vi "Cycle Duration Post Sub Steps types.vi"(10 "Cycle Duration Data in":T1, 11 "Sequence Context In":refnum<k7>) -> (0 "error out":errorcluster, 2 "Cycle Duration Data out":T1, 3 "Report Text":string)   [LabVIEW 2023, in "LTT_TeststandSteptypes.lvlib"]
uses:
  LTT_TeststandSteptypes.lvlib
  Control/Cycle Duration Data.ctl
  Control/Cycle Duration Selection.ctl
  HardwareAbstractionLayer_LVOOP/Report/Report_class/Control/Action FGV.ctl
  HardwareAbstractionLayer_LVOOP/Report/Report_class/Control/All Log Details.ctl
  HardwareAbstractionLayer_LVOOP/Report/Report_class/Control/UUT Test Info.ctl
  HardwareAbstractionLayer_LVOOP/Report/Report_class/Control/FE FRAME LOG.ctl
  HardwareAbstractionLayer_LVOOP/Report/Report_class/Control/FF FRAME LOG.ctl
  HardwareAbstractionLayer_LVOOP/Report/Report_class/Control/LIMIT TABLE.ctl
  HardwareAbstractionLayer_LVOOP/Report/Report_class/Control/ERROR LOG APPEND.ctl
  HardwareAbstractionLayer_LVOOP/Report/Report_class/Control/ERROR LOG.ctl
  HardwareAbstractionLayer_LVOOP/Report/Report_class/Control/FA FRAME LOG.ctl
  HardwareAbstractionLayer_LVOOP/Report/Report_class/Control/TEST RESULT LOG APPEND.ctl
  HardwareAbstractionLayer_LVOOP/Report/Report_class/Control/TEST RESULT LOG.ctl
  HardwareAbstractionLayer_LVOOP/Report/Report_class/Control/SYSTEM LOG.ctl
  HardwareAbstractionLayer_LVOOP/Report/Report_class/Control/Temperature LOG.ctl
  HardwareAbstractionLayer_LVOOP/Report/Report_class/Control/POWER STATUS.ctl
  HardwareAbstractionLayer_LVOOP/Report/Report_class/Control/CYCLE_DURATION_LOG.ctl
  HardwareAbstractionLayer_LVOOP/Database/SQL Public VI/Control/DB Options.ctl
  HardwareAbstractionLayer_LVOOP/Database/Database.lvclass
  HardwareAbstractionLayer_LVOOP/Report/Report_class/Report.lvclass
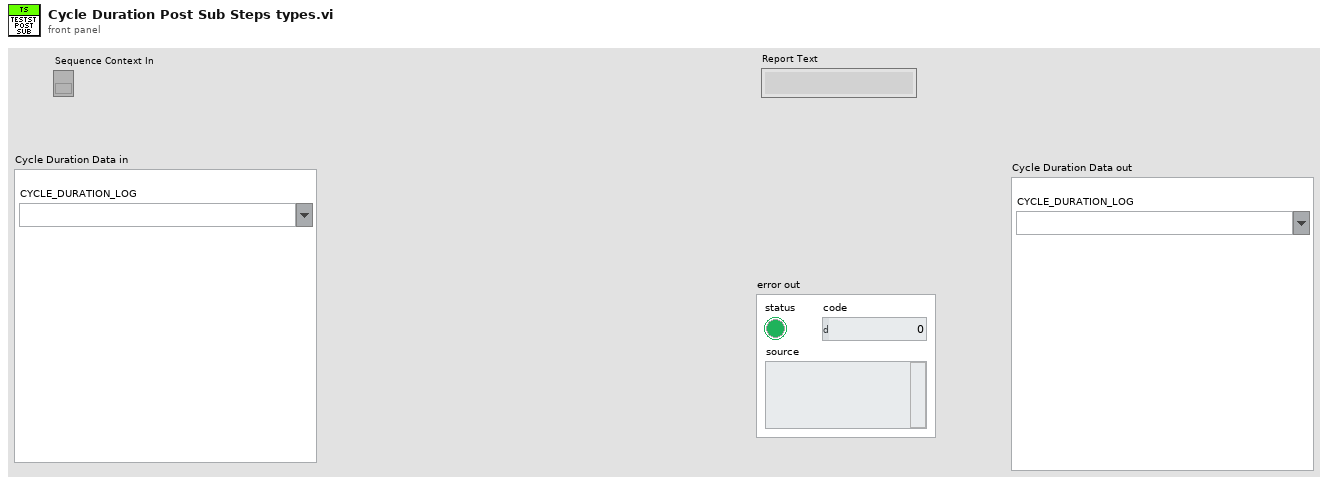
[diagram p1: front panel]
types:
  T1 = typedef "LTT_TeststandSteptypes.lvlib/Cycle Duration Data.ctl" = cluster{"CYCLE_DURATION_LOG":T2}
  T2 = typedef "LTT_TeststandSteptypes.lvlib/Cycle Duration Selection.ctl" = string
  T3 = typedef "HardwareAbstractionLayer_LVOOP.lvlib/Report.lvclass/Action FGV.ctl" = enum16{"Init", "Set Project Name", "Set Product Name", "Set Product Varient", "Set Test Name", "Set Test Phase", "Set Test Description", "Set Temp Chamber Name", "Set Cycle Duration", "Set Current Cycle Number", "Set Schema", "Set Total No Of Cycle", "Set Current Test Mode", "Set All Data", "Get All Data"}
  T4 = typedef "HardwareAbstractionLayer_LVOOP.lvlib/Report.lvclass/Result FGV Data.ctl" = cluster{"Project Name":string, "Product Name":string, "Product Varient":string, "Test Name":string, "Test Phase":string, "Test Description":string, "Temp Chamber Name":string, "Schema":string, "Total No of Cycles":u32, "Current Cycle Number":u32, "Cycle Duration":u32, "Current Test Mode":string}
  T5 = typedef "HardwareAbstractionLayer_LVOOP.lvlib/Report.lvclass/All Log Details.ctl" = cluster{"UUT_TEST_INFO":T6, "FE_FRAME_LOG":T7, "FF_FRAME_LOG":T8, "LIMIT_TABLE":T9, "ERROR LOG Append":T10, "FA_FRAME_LOG":T12, "Socket No":u16, "TEST RESULT LOG Append":T13, "SYSTEM_LOG":T15, "Temperature log":T16, "POWER_STATUS":T17, "CYCLE_DURATION_LOG":T18}
  T6 = typedef "HardwareAbstractionLayer_LVOOP.lvlib/Report.lvclass/UUT Test Info.ctl" = cluster{"ID":string, "STATION_ID":string, "TEST_SOCKET_INDEX":string, "UUT_SERIAL_NUMBER":string, "TSW_VER":string, "VAL_SW_VER":string, "PROJECT_NAME":string, "PRODUCT_NAME":string, "PRODUCT_VARIANT":string, "TEST_NAME":string, "TEST_PHASE":string, "TEST_DESCRIPTION":string, "TEMP_CHAMBER_NAME":string, "START_DATE_TIME":string, "STOP_DATE_TIME ":string, "START_CYCLE_COUNT":string, "STOP_CYCLE_COUNT":string, "EXECUTION_TIME":string, "UUT_STATUS":string, "UUT_ERROR_CODE":string, "UUT_ERROR_MESSAGE":string, "TEST_SEQUENCE":string}
  T7 = typedef "HardwareAbstractionLayer_LVOOP.lvlib/Report.lvclass/FE FRAME LOG.ctl" = cluster{"ID":string, "UUT_TEST_INFO":string, "DATE_TIME":string, "CYCLE_NUMBER":string, "TEST_MODE":string, "CHAMBER_TEMP":string, "CAN_FRAME_RX":string, "Test Mode":u32, "LV_PPS_VOLTAGE":string, "LV_PPS_CURRENT":string, "HV_PPS_VOLTAGE":string, "HV_PPS_CURRENT":string, "SOCKET_NUMBER":string, "CAN_FRAME_RX_NO_OFF_BYTE":string}
  T8 = typedef "HardwareAbstractionLayer_LVOOP.lvlib/Report.lvclass/FF FRAME LOG.ctl" = cluster{"ID":string, "UUT_TEST_INFO":string, "DATE_TIME":string, "CYCLE_NUMBER":string, "TEST_MODE":string, "CAN_FRAME_RX":string, "CHAMBER_TEMP":string, "TestMode":u32, "SOCKET_NUMBER":string, "CAN_FRAME_RX_NO_OFF_BYTE":string}
  T9 = typedef "HardwareAbstractionLayer_LVOOP.lvlib/Report.lvclass/LIMIT TABLE.ctl" = cluster{"ID":string, "PRODUCT_NAME":string, "PRODUCT_VARIANT":string, "TEST_MODE":string, "PARAMETER_NAME":string, "COMPARISON_TYPE":string, "LOW_LIMIT":string, "HIGH_LIMIT":string, "UNIT":string, "ERROR_MESSSAGE":string, "SEVERITY":string}
  T10 = typedef "HardwareAbstractionLayer_LVOOP.lvlib/Report.lvclass/ERROR LOG APPEND.ctl" = T11[]
  T11 = typedef "HardwareAbstractionLayer_LVOOP.lvlib/Report.lvclass/ERROR LOG.ctl" = cluster{"ID":string, "UUT_TEST_INFO":string, "DATE_TIME":string, "CYCLE_NUMBER":string, "TEST_MODE":string, "SIGNAL_NAME":string, "SIGNAL_VALUE":string, "UNIT":string, "COMPARISON_VALUE":string, "ERROR_MESSAGE":string, "FRAME_TYPE":string, "LIMITID":string, "SOCKET_NUMBER":string}
  T12 = typedef "HardwareAbstractionLayer_LVOOP.lvlib/Report.lvclass/FA FRAME LOG.ctl" = cluster{"UUT_TEST_INFO":string, "CAN_FRAME_RX":string, "CAN_FRAME_RX_NO_OFF_BYTE":string}
  T13 = typedef "HardwareAbstractionLayer_LVOOP.lvlib/Report.lvclass/TEST RESULT LOG APPEND.ctl" = T14[]
  T14 = typedef "HardwareAbstractionLayer_LVOOP.lvlib/Report.lvclass/TEST RESULT LOG.ctl" = cluster{"ID":string, "UUT_TEST_INFO":string, "DATE_TIME":string, "CYCLE_NUMBER":string, "TEST_MODE":string, "SIGNAL_NAME":string, "SIGNAL_VALUE":string, "COMPARISON_VALUE":string, "ERROR_MESSAGE":string, "FRAME_TYPE":string, "LIMITID":string, "TEST_RESULT":string, "SOCKET_NUMBER":string}
  T15 = typedef "HardwareAbstractionLayer_LVOOP.lvlib/Report.lvclass/SYSTEM LOG.ctl" = cluster{"ID ":string, "DATE_TIME":string, "CYCLE_NUMBER":string, "TEST_MODE":string, "ERROR_MESSAGE":string}
  T16 = typedef "HardwareAbstractionLayer_LVOOP.lvlib/Report.lvclass/Temperature LOG.ctl" = cluster{"TEST_MODE":string, "CYCLE_NUMBER":string, "TEMPERATURE":cluster{"LV_PPS_TEMPERATURE":dbl, "HV_PPS1_TEMPERATURE":dbl, "HV_PPS2_TEMPERATURE":dbl, "HV_PPS3_TEMPERATURE":dbl, "HV_PPS4_TEMPERATURE":dbl, "HV_PPS5_TEMPERATURE":dbl, "HV_PPS6_TEMPERATURE":dbl, "CHAMBER_TEMPERATURE":dbl, "LOAD_U1_TEMPERATURE":dbl, "LOAD_V1_TEMPERATURE":dbl, "LOAD_W1_TEMPERATURE":dbl, "LOAD_U2_TEMPERATURE":dbl, "LOAD_V2_TEMPERATURE":dbl, "LOAD_W2_TEMPERATURE":dbl, "LOAD_U3_TEMPERATURE":dbl, "LOAD_V3_TEMPERATURE":dbl, "LOAD_W3_TEMPERATURE":dbl}, "Temperature Inrange":cluster{"LVPPS_Trip?":bool, "HVPPS1_Trip?":bool, "HVPPS2_Trip?":bool, "HVPPS3_Trip?":bool, "HVPPS4_Trip?":bool, "HVPPS5_Trip?":bool, "HVPPS6_Trip?":bool, "Chamber_Trip?":bool}}
  T17 = typedef "HardwareAbstractionLayer_LVOOP.lvlib/Report.lvclass/POWER STATUS.ctl" = cluster{"TEST_MODE":string, "CYCLE_NUMBER":string, "TYPE_POWER":string, "STATE":string}
  T18 = typedef "HardwareAbstractionLayer_LVOOP.lvlib/Report.lvclass/CYCLE_DURATION_LOG.ctl" = cluster{"CYCLE_NUMBER":string}
  T19 = typedef "HardwareAbstractionLayer_LVOOP.lvlib/Database.lvclass/DB Options.ctl" = enum16{"Init", "Select Data", "Insert Data", "Update Data", "Delete Data", "Execute Query", "Create Schema", "Create Table", "List Tables", "List Columns", "Close"}
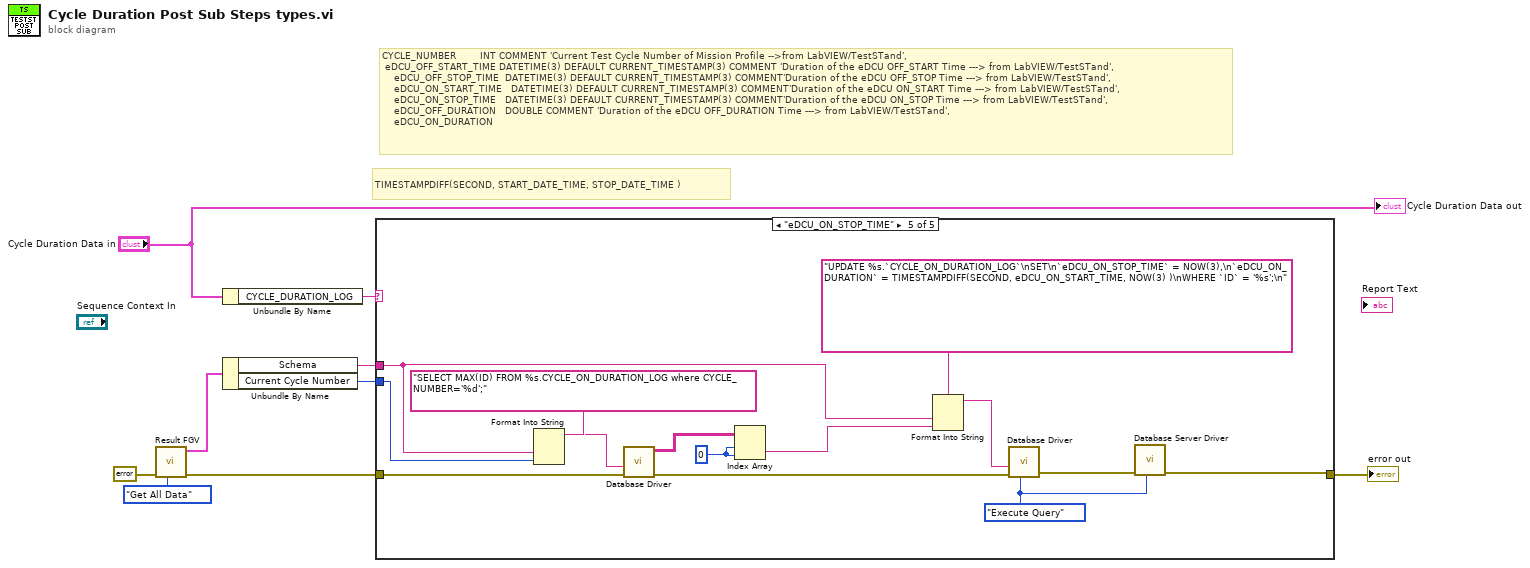
[diagram p0: block diagram]
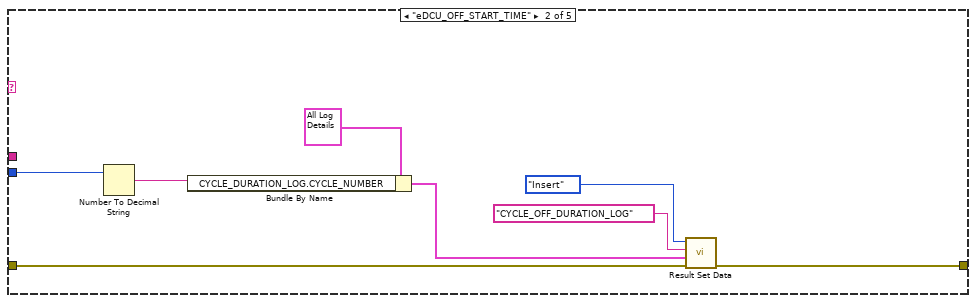
[diagram p3: hidden frame]
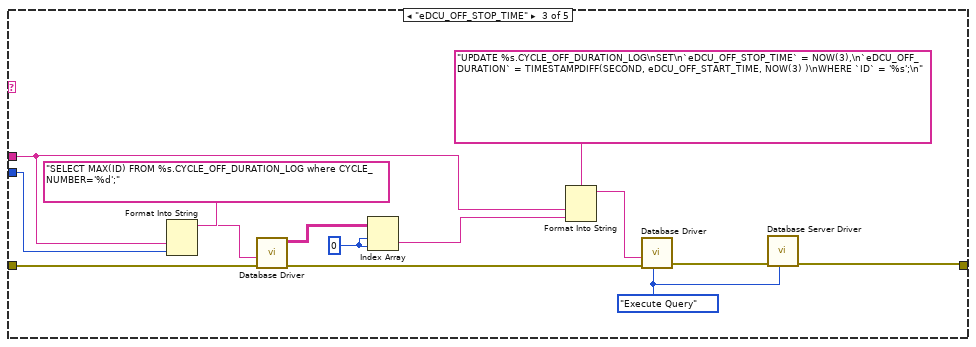
[diagram p4: hidden frame]
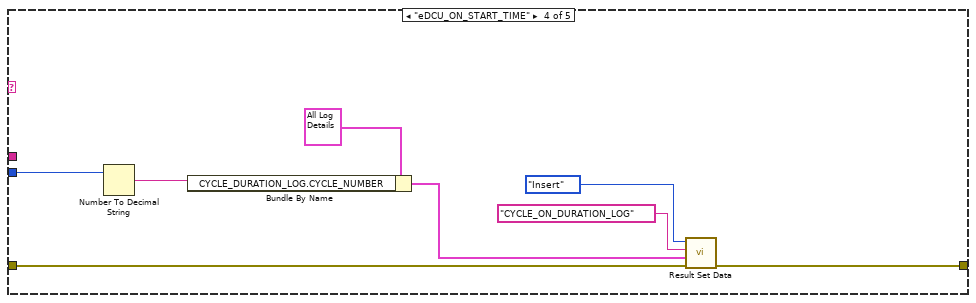
[diagram p5: hidden frame]
diagram:
  # "CYCLE_NUMBER        INT COMMENT 'Current Test Cycle Number of Mission Profile -->from LabVIEW/TestSTand',\n\teDCU_OFF_START_TIME DATETIME(3) DEFAULT CURRENT_TIMESTAMP(3) COMMENT 'Duration of the eDCU OFF_START Time ---> from LabVIEW/TestSTand',\n    eDCU_OFF_STOP_TIME  DATETIME(3) DEFAULT CURRENT_TIMESTAMP(3) COMMENT'Duration of the eDCU OFF_STOP Time ---> from LabVIEW/TestSTand',\n    eDCU_ON_START_TIME   DATETIME(3) DEFAULT CURRENT_TIMESTAMP(3) COMMENT'Duration of the eDCU ON_START Time ---> from LabVIEW/TestSTand',\n    eDCU_ON_STOP_TIME   DATETIME(3) DEFAULT CURRENT_TIMESTAMP(3) COMMENT'Duration of the eDCU ON_STOP Time ---> from LabVIEW/TestSTand',\n    eDCU_OFF_DURATION   DOUBLE COMMENT 'Duration of the eDCU OFF_DURATION Time ---> from LabVIEW/TestSTand',\n    eDCU_ON_DURATION"
  # "TIMESTAMPDIFF(SECOND, START_DATE_TIME, STOP_DATE_TIME )"
  n1 = call "Result FGV.vi"("Action(Get All Data)"=Action_FGV."Get All Data", "error in"=errorcluster {"status"=FALSE, "code"=0, "source"=""}) -> ("error out"=w2:errorcluster, "Result FGV Data Out"=w5:T4)  [unwired: 8 in]
  n2 = Unbundle By Name("Cycle Duration Data in") -> ("CYCLE_DURATION_LOG"=w8:T2)
  n3 = Unbundle By Name(w5) -> ("Schema"=w4:string, "Current Cycle Number"=w3:u32)
  n4 = case shown="\"eDCU_ON_STOP_TIME\"" w8 {
    tunnel: w4 -> [_ _ w19 _ w41]
    tunnel: w3 -> [_ w13 w30 w35 w52]
    tunnel: w2 -> [w10 w14 w32 w36 w54]
    tunnel: [w10 w11 w24 w33 w46] -> w1
    frame "", Default {
    }
    frame "eDCU_OFF_START_TIME" {
      n5 = Number To Decimal String(number=w13) -> (decimal integer string=w12:string)  [unwired: 1 in]
      n6 = Bundle By Name(cluster=T5 {"UUT_TEST_INFO"={"ID"="", "STATION_ID"="", "TEST_SOCKET_INDEX"="", "UUT_SERIAL_NUMBER"="", "TSW_VER"="", "VAL_SW_VER"="", "PROJECT_NAME"="", "PRODUCT_NAME"="", "PRODUCT_VARIANT"="", "TEST_NAME"="", "TEST_PHASE"="", "TEST_DESCRIPTION"="", "TEMP_CHAMBER_NAME"="", "START_DATE_TIME"="", "STOP_DATE_TIME "="", "START_CYCLE_COUNT"="", "STOP_CYCLE_COUNT"="", "EXECUTION_TIME"="", "UUT_STATUS"="", "UUT_ERROR_CODE"="", "UUT_ERROR_MESSAGE"="", "TEST_SEQUENCE"=""}, "FE_FRAME_LOG"={"ID"="", "UUT_TEST_INFO"="", "DATE_TIME"="", "CYCLE_NUMBER"="", "TEST_MODE"="", "CHAMBER_TEMP"="", "CAN_FRAME_RX"="", "Test Mode"=0, "LV_PPS_VOLTAGE"="", "LV_PPS_CURRENT"="", "HV_PPS_VOLTAGE"="", "HV_PPS_CURRENT"="", "SOCKET_NUMBER"="", "CAN_FRAME_RX_NO_OFF_BYTE"=""}, "FF_FRAME_LOG"={"ID"="", "UUT_TEST_INFO"="", "DATE_TIME"="", "CYCLE_NUMBER"="", "TEST_MODE"="", "CAN_FRAME_RX"="", "CHAMBER_TEMP"="", "TestMode"=0, "SOCKET_NUMBER"="", "CAN_FRAME_RX_NO_OFF_BYTE"=""}, "LIMIT_TABLE"={"ID"="", "PRODUCT_NAME"="", "PRODUCT_VARIANT"="", "TEST_MODE"="", "PARAMETER_NAME"="", "COMPARISON_TYPE"="", "LOW_LIMIT"="", "HIGH_LIMIT"="", "UNIT"="", "ERROR_MESSSAGE"="", "SEVERITY"=""}, "ERROR LOG Append"=[], "FA_FRAME_LOG"={"UUT_TEST_INFO"="", "CAN_FRAME_RX"="", "CAN_FRAME_RX_NO_OFF_BYTE"=""}, "Socket No"=1, "TEST RESULT LOG Append"=[], "SYSTEM_LOG"={"ID "="", "DATE_TIME"="", "CYCLE_NUMBER"="", "TEST_MODE"="", "ERROR_MESSAGE"=""}, "Temperature log"={"TEST_MODE"="", "CYCLE_NUMBER"="", "TEMPERATURE"={"LV_PPS_TEMPERATURE"=0.0, "HV_PPS1_TEMPERATURE"=0.0, "HV_PPS2_TEMPERATURE"=0.0, "HV_PPS3_TEMPERATURE"=0.0, "HV_PPS4_TEMPERATURE"=0.0, "HV_PPS5_TEMPERATURE"=0.0, "HV_PPS6_TEMPERATURE"=0.0, "CHAMBER_TEMPERATURE"=0.0, "LOAD_U1_TEMPERATURE"=0.0, "LOAD_V1_TEMPERATURE"=0.0, "LOAD_W1_TEMPERATURE"=0.0, "LOAD_U2_TEMPERATURE"=0.0, "LOAD_V2_TEMPERATURE"=0.0, "LOAD_W2_TEMPERATURE"=0.0, "LOAD_U3_TEMPERATURE"=0.0, "LOAD_V3_TEMPERATURE"=0.0, "LOAD_W3_TEMPERATURE"=0.0}, "Temperature Inrange"={"LVPPS_Trip?"=FALSE, "HVPPS1_Trip?"=FALSE, "HVPPS2_Trip?"=FALSE, "HVPPS3_Trip?"=FALSE, "HVPPS4_Trip?"=FALSE, "HVPPS5_Trip?"=FALSE, "HVPPS6_Trip?"=FALSE, "Chamber_Trip?"=FALSE}}, "POWER_STATUS"={"TEST_MODE"="", "CYCLE_NUMBER"="", "TYPE_POWER"="", "STATE"=""}, "CYCLE_DURATION_LOG"={"CYCLE_NUMBER"=""}} ("Set Data"), "CYCLE_DURATION_LOG.CYCLE_NUMBER"=w12) -> (w15:T5)
      n7 = call "Result Set Data.vi"("error in"=w14, "Set Data"=w15, "Table Name"="CYCLE_OFF_DURATION_LOG", "Action"=enum16{"Insert", "Update"}."Insert") -> ("error out"=w11:errorcluster)  [unwired: 7 in]
    }
    frame "eDCU_OFF_STOP_TIME" {
      w23 = DB_Options."Execute Query" ("Options")
      w25 = 0 ("index (row)")
      n8 = Format Into String(format string="SELECT MAX(ID) FROM %s.CYCLE_OFF_DURATION_LOG where CYCLE_NUMBER='%d';", w19, w30) -> (resulting string=w27:string)  [unwired: 2 in, 1 out]
      n9 = call "Database Driver.vi"("error in"=w32, "SQL query"=w27) -> ("error out"=w29:errorcluster, "data"=w26:string[][])  [unwired: 6 in, 2 out]
      n10 = Index Array(array=w26, index (row)=w25, index (col)=w25) -> (element=w20:string)
      n11 = Format Into String(format string="UPDATE %s.CYCLE_OFF_DURATION_LOG\nSET\n`eDCU_OFF_STOP_TIME` = NOW(3),\n`eDCU_OFF_DURATION` = TIMESTAMPDIFF(SECOND, eDCU_OFF_START_TIME, NOW(3) )\nWHERE `ID` = '%s';\n", w19, w20) -> (resulting string=w21:string)  [unwired: 2 in, 1 out]
      n12 = call "Database Driver.vi"("Options"=w23, "error in"=w29, "SQL query"=w21) -> ("error out"=w28:errorcluster)  [unwired: 5 in, 3 out]
      n13 = call "Database Server Driver.vi"("Options"=w23, "error in"=w28) -> ("error out"=w24:errorcluster)  [unwired: 6 in, 3 out]
    }
    frame "eDCU_ON_START_TIME" {
      n14 = Number To Decimal String(number=w35) -> (decimal integer string=w34:string)  [unwired: 1 in]
      n15 = Bundle By Name(cluster=T5 {"UUT_TEST_INFO"={"ID"="", "STATION_ID"="", "TEST_SOCKET_INDEX"="", "UUT_SERIAL_NUMBER"="", "TSW_VER"="", "VAL_SW_VER"="", "PROJECT_NAME"="", "PRODUCT_NAME"="", "PRODUCT_VARIANT"="", "TEST_NAME"="", "TEST_PHASE"="", "TEST_DESCRIPTION"="", "TEMP_CHAMBER_NAME"="", "START_DATE_TIME"="", "STOP_DATE_TIME "="", "START_CYCLE_COUNT"="", "STOP_CYCLE_COUNT"="", "EXECUTION_TIME"="", "UUT_STATUS"="", "UUT_ERROR_CODE"="", "UUT_ERROR_MESSAGE"="", "TEST_SEQUENCE"=""}, "FE_FRAME_LOG"={"ID"="", "UUT_TEST_INFO"="", "DATE_TIME"="", "CYCLE_NUMBER"="", "TEST_MODE"="", "CHAMBER_TEMP"="", "CAN_FRAME_RX"="", "Test Mode"=0, "LV_PPS_VOLTAGE"="", "LV_PPS_CURRENT"="", "HV_PPS_VOLTAGE"="", "HV_PPS_CURRENT"="", "SOCKET_NUMBER"="", "CAN_FRAME_RX_NO_OFF_BYTE"=""}, "FF_FRAME_LOG"={"ID"="", "UUT_TEST_INFO"="", "DATE_TIME"="", "CYCLE_NUMBER"="", "TEST_MODE"="", "CAN_FRAME_RX"="", "CHAMBER_TEMP"="", "TestMode"=0, "SOCKET_NUMBER"="", "CAN_FRAME_RX_NO_OFF_BYTE"=""}, "LIMIT_TABLE"={"ID"="", "PRODUCT_NAME"="", "PRODUCT_VARIANT"="", "TEST_MODE"="", "PARAMETER_NAME"="", "COMPARISON_TYPE"="", "LOW_LIMIT"="", "HIGH_LIMIT"="", "UNIT"="", "ERROR_MESSSAGE"="", "SEVERITY"=""}, "ERROR LOG Append"=[], "FA_FRAME_LOG"={"UUT_TEST_INFO"="", "CAN_FRAME_RX"="", "CAN_FRAME_RX_NO_OFF_BYTE"=""}, "Socket No"=1, "TEST RESULT LOG Append"=[], "SYSTEM_LOG"={"ID "="", "DATE_TIME"="", "CYCLE_NUMBER"="", "TEST_MODE"="", "ERROR_MESSAGE"=""}, "Temperature log"={"TEST_MODE"="", "CYCLE_NUMBER"="", "TEMPERATURE"={"LV_PPS_TEMPERATURE"=0.0, "HV_PPS1_TEMPERATURE"=0.0, "HV_PPS2_TEMPERATURE"=0.0, "HV_PPS3_TEMPERATURE"=0.0, "HV_PPS4_TEMPERATURE"=0.0, "HV_PPS5_TEMPERATURE"=0.0, "HV_PPS6_TEMPERATURE"=0.0, "CHAMBER_TEMPERATURE"=0.0, "LOAD_U1_TEMPERATURE"=0.0, "LOAD_V1_TEMPERATURE"=0.0, "LOAD_W1_TEMPERATURE"=0.0, "LOAD_U2_TEMPERATURE"=0.0, "LOAD_V2_TEMPERATURE"=0.0, "LOAD_W2_TEMPERATURE"=0.0, "LOAD_U3_TEMPERATURE"=0.0, "LOAD_V3_TEMPERATURE"=0.0, "LOAD_W3_TEMPERATURE"=0.0}, "Temperature Inrange"={"LVPPS_Trip?"=FALSE, "HVPPS1_Trip?"=FALSE, "HVPPS2_Trip?"=FALSE, "HVPPS3_Trip?"=FALSE, "HVPPS4_Trip?"=FALSE, "HVPPS5_Trip?"=FALSE, "HVPPS6_Trip?"=FALSE, "Chamber_Trip?"=FALSE}}, "POWER_STATUS"={"TEST_MODE"="", "CYCLE_NUMBER"="", "TYPE_POWER"="", "STATE"=""}, "CYCLE_DURATION_LOG"={"CYCLE_NUMBER"=""}} ("Set Data"), "CYCLE_DURATION_LOG.CYCLE_NUMBER"=w34) -> (w37:T5)
      n16 = call "Result Set Data.vi"("error in"=w36, "Set Data"=w37, "Table Name"="CYCLE_ON_DURATION_LOG", "Action"=enum16{"Insert", "Update"}."Insert") -> ("error out"=w33:errorcluster)  [unwired: 7 in]
    }
    frame "eDCU_ON_STOP_TIME" {
      w45 = DB_Options."Execute Query" ("Options")
      w47 = 0 ("index (row)")
      n17 = Format Into String(format string="SELECT MAX(ID) FROM %s.CYCLE_ON_DURATION_LOG where CYCLE_NUMBER='%d';", w41, w52) -> (resulting string=w49:string)  [unwired: 2 in, 1 out]
      n18 = call "Database Driver.vi"("error in"=w54, "SQL query"=w49) -> ("error out"=w51:errorcluster, "data"=w48:string[][])  [unwired: 6 in, 2 out]
      n19 = Index Array(array=w48, index (row)=w47, index (col)=w47) -> (element=w42:string)
      n20 = Format Into String(format string="UPDATE %s.`CYCLE_ON_DURATION_LOG`\nSET\n`eDCU_ON_STOP_TIME` = NOW(3),\n`eDCU_ON_DURATION` = TIMESTAMPDIFF(SECOND, eDCU_ON_START_TIME, NOW(3) )\nWHERE `ID` = '%s';\n", w41, w42) -> (resulting string=w43:string)  [unwired: 2 in, 1 out]
      n21 = call "Database Driver.vi"("Options"=w45, "error in"=w51, "SQL query"=w43) -> ("error out"=w50:errorcluster)  [unwired: 5 in, 3 out]
      n22 = call "Database Server Driver.vi"("Options"=w45, "error in"=w50) -> ("error out"=w46:errorcluster)  [unwired: 6 in, 3 out]
    }
  }
  "error out" <- w1
  "Cycle Duration Data out" <- "Cycle Duration Data in"
